vi "Record Instruments.vi"(8 "Error In":errorcluster, 11 "Instrument List in":T1[](array[typedef]) {"Status" format="%.0x"}) -> (0 "Error Out":errorcluster, 3 "Instrument List out":T1[](array[typedef]) {"Status" format="%.0x"})   [LabVIEW 2020]
doc: "Record all found instruments as unique strings in TSV text file. Upload all Instrument files to server.\n(c) Scott Hannahs, September 2019\n<sth@magnet.fsu.edu>"
uses:
  New NML Data Acq/Sub Controls/Instrument IDN.ctl
  <vilib>/Utility/file.llb/Read Delimited Spreadsheet (string).vi
  <vilib>/Utility/file.llb/Write Delimited Spreadsheet (string).vi
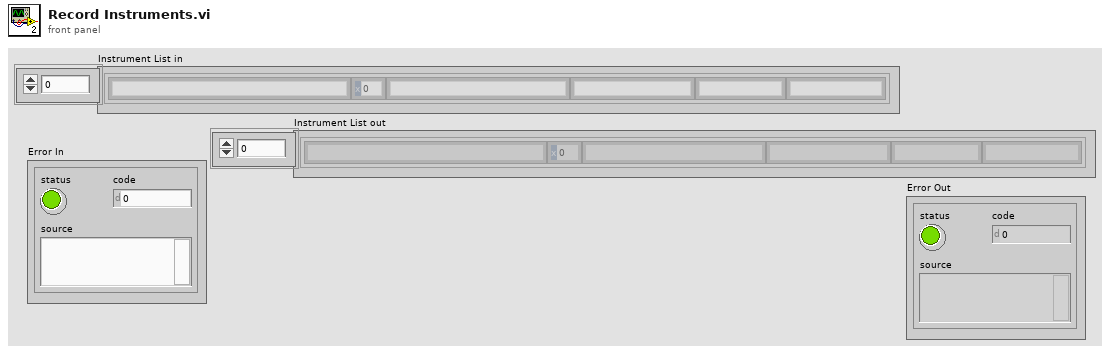
[diagram p1: front panel]
types:
  T1 = typedef "Instrument IDN.ctl" = cluster{"VISA Address":string, "Status":u16, "Manufacturer":string, "Model":string, "Info":string, "Info 2":string, "Misc Data":variant}
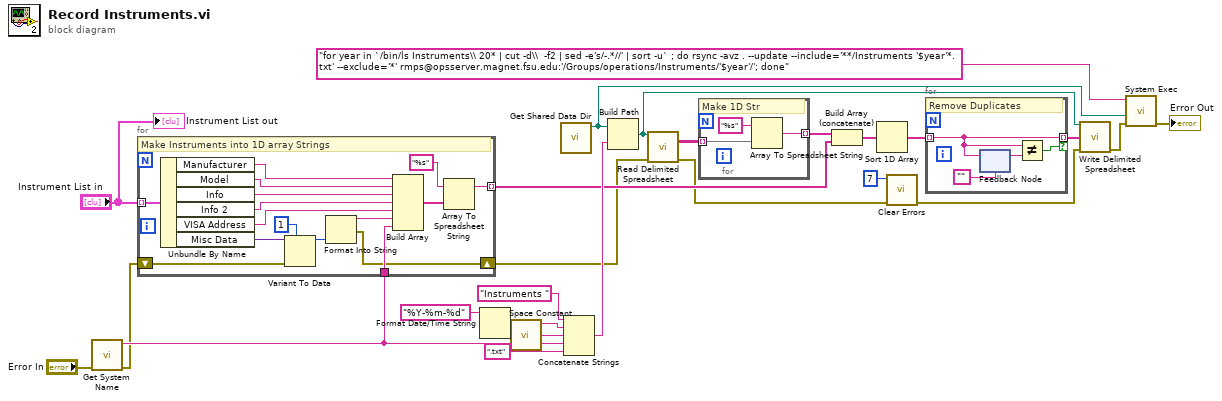
[diagram p0: block diagram]
diagram:
  n1 = call "Get System Name.vi"("Error In"="Error In") -> ("Error Out"=w2:errorcluster, "System Name"=w23:string)  [unwired: 4 in, 1 out]
  n2 = for {
    tunnel: "Instrument List in" -> [w41] mode=indexing
    tunnel: [w28] -> w17 mode=indexing
    tunnel: w23 -> [w35]
    shift-right: [w29] -> w9
    shift-left: w2 -> [w30]
    # "Make Instruments into 1D array Strings"
    n3 = Unbundle By Name(w41) -> ("Manufacturer"=w40:string, "Model"=w39:string, "Info"=w38:string, "Info 2"=w37:string, "VISA Address"=w36:string, "Misc Data"=w33:variant)
    n4 = Variant To Data(error in=w30, type=1, Variant=w33) -> (data=w34:i32)  [unwired: 1 out]
    n5 = Format Into String(w34) -> (resulting string=w31:string, error out=w29:errorcluster)  [unwired: 3 in]
    n6 = Build Array(w40, w39, w38, w37, w36, w31, w35) -> (w27:string[])
    n7 = Array To Spreadsheet String(array=w27, 3:"%s" ("format string")) -> (spreadsheet string=w28:string)  [unwired: 1 in]
  }
  n8 = Format Date/Time String(time format string (%c)="%Y-%m-%d") -> (date/time string=w22:string)  [unwired: 2 in]
  n9 = call <vilib>:"Space Constant.vi"() -> ("String"=w21:string)
  n10 = call "Get Shared Data Dir.vi"() -> ("Data Directory Path"=w7:path)  [unwired: 2 in, 1 out]
  n11 = Concatenate Strings("Instruments " ("string"), w22, w21, w23, ".txt" ("string")) -> (w18:string)
  n12 = Build Path(base path=w7, name or relative path=w18) -> (appended path=w6:path)
  n13 = call-poly <vilib>:"Read Delimited Spreadsheet.vi"("file path (dialog if empty)"=w6, "error in (no error)"=w9) -> ("all rows"=w15:string[][], "error out"=w5:errorcluster)  [unwired: 8 in, 4 out]
  n14 = for {
    tunnel: w15 -> [w44] mode=indexing
    tunnel: [w42] -> w14 mode=indexing
    # "Make 1D Str"
    n15 = Array To Spreadsheet String(array=w44, 3:"%s" ("format string")) -> (spreadsheet string=w42:string)  [unwired: 1 in]
  }
  n16 = Build Array (concatenate)(w14, w17) -> (w16:string[])
  n17 = Sort 1D Array(array=w16) -> (sorted array=w13:string[])
  n18 = call <vilib>:"Clear Errors.vi"("error in (no error)"=w5, "specific error code to clear (0: all)"=7) -> ("error out"=w4:errorcluster)  [unwired: 4 in, 1 out]
  n19 = for {
    tunnel: w13 -> [w47] mode=indexing
    tunnel: [w47] -> w12 mode=indexing if=w48
    # "Remove Duplicates"
    n20 = feedback-in #1(w47) -> ()
    n21 = feedback #1("") -> (w46:string)
    n22 = Not Equal?(x=w47, y=w46) -> (x != y?=w48:bool)
  }
  n23 = call-poly <vilib>:"Write Delimited Spreadsheet.vi"("file path (dialog if empty)"=w6, "1D data"=w12, "error in (no error)"=w4) -> ("error out"=w10:errorcluster)  [unwired: 11 in, 1 out]
  n24 = call <vilib>:"System Exec.vi"("error in (no error)"=w10, "working directory"=w7, "command line"="for year in `/bin/ls Instruments\\ 20* | cut -d\\  -f2 | sed -e's/-.*//' | sort -u` ; do rsync -avz . --update --include='**/Instruments '$year'*.txt' --exclude='*' rmps@opsserver.magnet.fsu.edu:'/Groups/operations/Instruments/'$year'/'; done") -> ("error out"=→"Error Out":errorcluster)  [unwired: 5 in, 3 out]
  "Instrument List out" <- "Instrument List in"
